vi "AlliGator Phasor Plot ROI Manager.vi"() -> ()   [LabVIEW 2021, in "AlliGator ROIs.lvlib"]
doc: "Phasor Plot image ROI list display UI."
uses:
  AlliGator ROIs.lvlib
  AlliGator ROI Manager Actions.ctl
  AlliGator Refnums List.ctl
  Image/Image Control Refnum.ctl
  Image/Image Display Event.ctl
  <vilib>/Utility/miscctls.llb/LVPoint32TypeDef.ctl
  AlliGator Variables List.ctl
  Image/Named ROI Description.ctl
  Variant/Variant to Data/Variant to String.vi
  AlliGator Phasor Plot Image ROI Storage [SGL] v3.vi
  AlliGator Globals, Variables & Constants.lvlib
  Image/Image.lvlib
  AlliGator Action Engine.lvlib
  Notebook/Notebook.lvlib
  AlliGator Notebook.lvlib
  Variant/Variant to Data/Variant to Data.lvlib
  AlliGator Phasor Plot.lvlib
  Rich Text Box/Rich Text Box.lvlib
panel:
  in  "ROI List":i32(listbox)
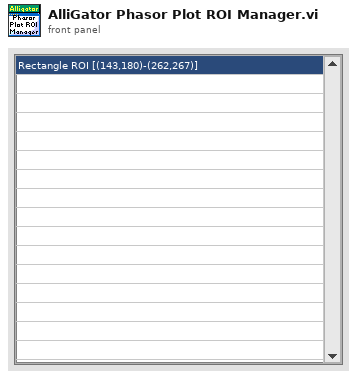
[diagram p1: front panel]
types:
  T1 = typedef "Image.lvlib/Image Control Refnum.ctl" = refnum<vi>
  T2 = typedef "AlliGator Globals, Variables & Constants.lvlib/AlliGator Refnums List.ctl" = enum16{"---------- AlliGator Controls ----------", "AlliGator Tab Control Refnum", "---------- AlliGator Indicators ----------", "Source Image Display Refnum", "Phasor Plot Display Refnum", "Decay Fit Parameter Map Refnum", "---------- AlliGator VIs ----------", "AlliGator Settings Refnum", "AlliGator Launcher Refnum"}
  T3 = typedef "AlliGator ROIs.lvlib/AlliGator ROI Manager Actions.ctl" = enum16{"Undefined", "Delete Current ROI", "Delete All Unselected ROIs", "Delete Multiple ROIs", "Delete All ROIs", "Swap ROIs", "Insert ROI", "Update Current ROI Descriptor", "Rename Current ROI", "Store New ROI", "Store Multiple ROIs", "Select Next ROI", "Select Previous ROI", "Find Selected ROI", "Show All ROIs", "Update ROI Manager Window", "Merge All ROIs", "Unmerge ROI", "Set Selected ROI by ID"}
  T4 = typedef "AlliGator ROIs.lvlib/AlliGator Image ROI Event refnum.ctl" = refnum<user-event>
  T5 = typedef "ROI Descriptor" = cluster{"Global Rectangle":i32[], "Contours":cluster{"ID":enum32{"External", "Internal"}, "Type":u32, "Coordinates":i32[]}[]}
  T6 = typedef "Image.lvlib/Image Display Event.ctl" = cluster{"Item Tag":string, "Image Control Refnum":T1, "Coords":T7, "Item Path":string}
  T7 = typedef "LVPoint32TypeDef.ctl" = cluster{"Horizontal":i32, "Vertical":i32}
  T8 = typedef "AlliGator Globals, Variables & Constants.lvlib/AlliGator Variables List.ctl" = enum16{"---- GUI ----", "Initialization Status", "State Indicators Refnum", "Original AlliGator Menu Items", "Current Action Loop State", "Script in progress", "Playback", "Loop Playback", "Search ROI Used", "Search ROI", "Decay Graph Max Legend Size", "Intensity Graph Max Legend Size", "Decay Statistics Graph Max Legend Size", "Phasor Graph Max Legend Size", "Phasor Ratio Graph Max Legend Size", "Lifetime Graph Max Legend Size", "---- Files ----", "Export Dataset Frames as Individual Files", "Show Batch Export Help Balloons", "Frames in Dataset", "ptu File Frame Start Indices", "Current Frame in Dataset", "Current Frame Timestamp", "------ Python Plugins ------", "Python Plugins Information", "Python Session", "Valid Python Session?", "---- Source Image ----", "Dataset Loaded", "Dataset Metadata", "Dataset Channel", "Dataset Data Description", "Background Dataset Metadata", "Background Dataset Channel", "Background Dataset Data Description", "Background File Subtraction", "Background File Path", "Background File Pile-up Correction", "Background File Pixel Well Capacity", "Background File Scaling Factor", "Source Image ROIs", "Current Source Image ROI", "Source Image ROI Event Refnum", "X_Source Image Display Range", "X_Source Image Palette Information", "Source Image Palette List", "Source Image Scale", "Current Dataset Load Settings", "Source Image:ROI Overlay Color", "---- Image Profile Window ----", "Image Profile:Overlay ROI in Source Image", "Image Profile Window Event Refnum", "Image Profile:IntensityType", "Image Profile:Intensity Average Type", "Image Profile:Intensity-weighted SDV", "Image Profile:Box Profile Type", "Image Profile Window Open", "Image Profile:Plotted Fit Parameter", "X_Type of Displayed Image", "X_Time Gate Slider", "Dataset Path", "Source Image Overlay to Erase", "Is Displayed Image Accumulated", "White Light Image Modified", "Mask Image Modified", "Macrotime Gate Separation", "------ Phasor Graph -------", "Phasor Graph:Show Line", "---- Phasor Plot ---", "Phasor Plot Parameters Changed", "FLI Dataset Modified since last Phasor Plot Calculation", "Phasor Harmonics Data", "Selected Phasor Harmonics", "Phasor Harmonic Manager Event Refnum", "Phasor Plot ROIs", "Current Phasor Plot ROI", "Phasor Plot ROI Event Refnum", "Phasor Plot Image Reference Points", "Phasor Plot Computed", "Phasor Plot Palette Information", "Phasor Plot Palette List", "Phasor Ratio Palette Information", "Phasor Ratio Palette List", "Phasor Image Scale", "Phasor Plot Image Overlay to Erase", "Phasor Plot Image Elements to Update", "Current Phasor Plot Calculation Parameters", "Current Phasor Calibration Options", "Reset Cumulated Phasor Plot", "Phasor Ratio Reference 1", "Phasor Ratio Lifetime Reference 1", "Phasor Ratio Reference 1 Frequency", "Phasor Ratio Reference 2", "Phasor Ratio Lifetime Reference 2", "Phasor Ratio Reference 2 Frequency", "---- Decay Analysis ----", "Number of Selected Decays to Fit", "LS Fit Results", "LAR Fit Results", "BS Fit Results", "Last Decay Max - Min", "Best Fit Parameters", "Best Fit Parameter Names", "Actual Size X", "Actual Size Y", "Binning X", "Binning Y", "Actual # Gates", "Dataset Number", "Gates to...", "Gates Skipped", "Gates to keep", "Gate Step", "Gate Separation", "Reversed Gates", "Pile-up Correction", "Pixel Well Capacity", "Background Subtracted", "Background Subtraction Method", "Background Definition Range", "Background File (deprecated)", "Number of Dataset Accumulated", "Array of Accumulated Dataset Paths", "Do Averaged Datasets", "Destination File Path", "Process Plot Target", "Use 1/D as Phasor Frequency", "---- Decay Fit Parameter Map -----", "Decay Fit Parameter Map Palette Information", "Decay Fit Parameter Map Palette List", "Local Decay Graph Window Event Refnum", "------- Local Decay Window ---------", "Use normalized IRF for convolution", "----- Miscellaneous ----", "Skippable Dialog Windows Status"}
  T9 = typedef "Image.lvlib/Named ROI Description.ctl" = cluster{"ROI Descriptor":T5, "ROI Name":string, "Overlay Color":u32}
  T10 = cluster{"data name":string, "drag data":variant}[]
  T11 = typedef "AlliGator Action Engine.lvlib/AlliGator Q Element.ctl" = cluster{"AlliGator Q Event":T12, "Data":variant}
  T12 = typedef "AlliGator Action Engine.lvlib/AlliGator Q Event.ctl" = enum16{"---- Files ----", "Files:Set Batch Export Files To Save", "Files:Set Dataset Loading & Pre-processing Options", "Files:Check #Frames in Dataset", "Files:Increment Frame Index", "Files:Open Mask Image", "Files:Open White Light Image", "Files:Open Single Dataset", "Files:New Folder of Folders Selected", "Files:Load File (all Types)_Scriptable", "Files:Move Flattened Series to Folders Series", "Files:Select Folder", "Files:Load FLI Dataset", "Files:Load Swiss SPAD 1 Dataset", "Files:Load Swiss SPAD 2 Dataset", "Files:Load .sdt FLI Dataset", "Files:Load .ptu FLI Dataset", "Files:Load .bin FLI Dataset", "Files:Load Single Gate Image Folder", "Files:Load I/m/phi Dataset (deprecated)", "Files:Load Single Image", "Files:Subtract Background File", "Files:Export FLI Dataset", "Files:Load HDF5 FLI Dataset", "Files:Set Destination File Path", "Files:Save Mask Image", "Files:Batch Conversion", "Files:New Folder Selected", "Files:Close FLI Dataset", "Files:Close FLI Dataset Series", "Files:Close White Light Image", "Files:Close Mask Image", "---- FLI Dataset ----", "FLI Dataset:Channel Arithmetic", "FLI Dataset:Export Average Lifetime Map as ASCII", "FLI Dataset:Export User-Defined Quantity Map as ASCII", "FLI Dataset:Python Function FLI Dataset Event", "FLI Dataset:ROI Analysis", "FLI Dataset:Tilted Logistic Square Gated IRF Characteristics Map", "FLI Dataset:Logistic Square Gated IRF Characteristics Map", "FLI Dataset:Square Gated IRF Characteristics Map", "FLI Dataset:Multi-ROI Single-Pixel Phasor Analysis", "FLI Dataset:Multi-ROI Single-Pixel NLSF Analysis", "FLI Dataset:All ROIs IRF Extraction", "FLI Dataset:All ROIs Decay Fit Non-Interactive (Fast + Individual IRF)", "FLI Dataset:All ROIs Phasor Analysis", "FLI Dataset:All ROIs Decay Fit", "FLI Dataset:Fluorescence Decay Statistics", "FLI Dataset:Update Decay Statistics Graph", "FLI Dataset:Get Decay from ROI", "FLI Dataset:All ROIs Average Lifetimes", "---- FLI Dataset Series ----", "FLI Dataset Series:Sum All Datasets in Series", "FLI Dataset Series:Add Dataset to Accumulated Dataset", "FLI Dataset Series:Display Accumulated Dataset", "FLI Dataset Series:Clear Dataset Series Sum", "FLI Dataset Series:Time-Series Analysis (NLSF)", "FLI Dataset Series:Time-Series Analysis (Phasor)", "---- Image ----", "Image:Update Image Profile Plots", "Image:Image Histogram Cursor Move", "Image:Image Histogram", "Image:Image Contrast", "Image:Set Image Histogram Cursor Move Flag", "Image:Clear Image Overlay", "Image:Use ROI as Search Area", "Image:Set ROI Diameter", "Image:Save Image Data as TIFF", "Image:Save Displayed Image with Overlay", "Image:Save Image Overlay Only", "Image:Save Image as Hot Pixel Mask", "Image:Change Source Image Color Palette", "Image:Copy Image to Clipboard", "Image:Source Image ROI Selection", "Image:Delete All ROIs", "Image:Delete All Unselected ROIs", "Image:Delete ROI", "Image:Merge All ROIs", "Image:Store ROI", "Image:Source Image ROI Storage", "Image:Export ROI Description to Notebook", "Image:Save ROI", "Image:Load ROI", "Image:Paste ROI Definition", "Image:Clear ROI", "Image:Identify ROIs in Mask Image", "Image:Create Complementary ROI", "Image:Create Contour ROI", "Image:Create ROI(s) from Pixels with Peak above Min_Scriptable", "Image:Create ROI(s) from Pixels with Intensity above Min_Scriptable", "Image:Compute ROI Statistics", "Image:Delete ROI(s) based on ROI Characteristics", "Image:Create ROI Grid", "Image:ROI to Individual Pixel ROIs", "Image:Python Function Source Image Event", "Image:Show Phasor Calibration Map ROI Centers", "Image:Convert ROI to Mask Image", "Image:Mouse Move", "Image:Mouse Up", "Image:Set Source Image Mouse Move Flag", "Image:Add Scale Bar Overlay", "Image:Delete Existing ROIs Option", "---- Decay ----", "Decay:Clear IRF/Reference Plot", "Decay:Clear Local IRFs", "Decay:Add Decay to Graph", "Decay:Smoothen Plot", "Decay:Smoothen Plot Tail", "Decay:Average Selected Plots", "Decay:Extract IRF", "Decay:Optimal IRF Extraction", "Decay:Threshold IRF", "Decay:Fit to Model IRF", "Decay:Fit IRF to Square Gate", "Decay:Fit IRF to Logistic Square Gate", "Decay:Fit IRF to Tilted Logistic Square Gate", "Decay:Create Bounding Cursors Set", "Decay:Export Bounding Cursors Definition to Notebook", "Decay:Denoise Plot", "Decay:Compute Cumulative Function", "Decay:Use as Reference Decay", "Decay:Show Reference Decay/IRF", "Decay:Extrapolate Decay", "Decay:Create Head & Tail Bounding Cursors", "Decay:Store Cursor-defined Head & Tail Fractions", "Decay:Rebin Plot", "Decay:1-Normalize Decay", "Decay:[0-1]-Normalize Plot", "Decay:Straighten Decay", "Decay:Shift Decay", "Decay:Fold Decay", "Decay:Fit Decay", "Decay:Global Fit of Selected Decays", "Decay:Post Global Fit Script", "Decay:Add Global Fit Parameters to Graph", "Decay:Add Decay Parameter(s) to Plot (Graph)", "Decay:Export Decay to Phasor Graph", "Decay:Plot Decay Shifts", "Decay:Compute Average Lifetime", "Decay:Plot Convolution", "Decay:Graph Tip Strip Update", "---- Decay Statistics ----", "Decay Statistics:Tip Strip Update", "---- Intensity Time Trace ----", "Intensity Time Trace:Use File Timestamp", "Intensity Time Trace:Load Intensity Corrections File", "Intensity Time Trace:Clear Intensity Corrections File", "Intensity Time Trace:Tip Strip Update", "---- Phasor Plot ----", "Phasor Plot:Build Phasor Plot", "Phasor Plot:Change Phasor Plot Color Palette", "Phasor Plot:Adjust Phasor Plot Display Range", "Phasor Plot:Highlight Image ROI in Phasor Plot", "Phasor Plot:Save Phasor Plot Image with Overlay", "Phasor Plot:Export Complex Phasor Map", "Phasor Plot:Export Phasor Ratio Map", "Phasor Plot:Export Average Lifetime Map", "Phasor Plot:Compute Phase Lifetime Histogram", "Phasor Plot:Compute Phasor Ratio Histogram", "Phasor Plot:Compute Phase Lifetime vs Intensity Scatter Plot", "Phasor Plot:Weber 2-Component Decomposition", "Phasor Plot:Update Phasor Color Map Vertices", "Phasor Plot:Clear Phasor Overlay", "Phasor Plot:Use Segment Extremities as References", "Phasor Plot:Use UC/Segment Intersections as References", "Phasor Plot:Use UC/Principal Axis Intersections as References", "Phasor Plot:Use UC/Linear Fit Intersections as References", "Phasor Plot:Update Phasor Plot Reference", "Phasor Plot:Show Local Phasor Info in Phasor Plot", "Phasor Plot:Update Phasor Plot State", "Phasor Plot:Phasor Plot ROI Storage", "Phasor Plot:Phasor Plot ROI Selection", "Phasor Plot:Python Function Phasor Plot Event", "Phasor Plot:Overlay Phasor ROI, Ratio or Map in Source Image", "Phasor Plot:Compute Decay of Selected Phasors", "Phasor Plot:Phasor at Image Pixel", "Phasor Plot:Mouse Move", "Phasor Plot:Mouse Up", "Phasor Plot:Display Range Mouse Move", "Phasor Plot:Set Mouse Move Flag", "---- Phasor Graph ----", "Phasor Graph:Calibrated Phasor Map Series", "Phasor Graph:Whole Image Phasor Scatter Plot (Todo)", "Phasor Graph:Get Phasor Value", "Phasor Graph:Create New Phasor Plot Dialog", "Phasor Graph:Update Last Phasor Value", "Phasor Graph:Update Phasor (m, phi)", "Phasor Graph:Remove Single Phasor from Plot", "Phasor Graph:Add Single Phasor to Plot", "Phasor Graph:Remove Phasor Plot", "Phasor Graph:Remove Selected Phasor Plots", "Phasor Graph:Clear Phasor Data", "Phasor Graph:Clear Phasor Graph", "Phasor Graph:Cursor Move", "Phasor Graph:Draw Cursor Connecting Line", "Phasor Graph:Clear Cursor Connecting Line", "Phasor Graph:Find UC Intersection", "Phasor Graph:Use UC/Cursor-Defined Line Intersections", "Phasor Graph:Use Selected Plots Fitted Line/UC Intersections", "Phasor Graph:Use Selected Plots Principal Axis/UC Intersections", "Phasor Graph:Show Single Phasor", "Phasor Graph:Save Single Phasor Plot", "Phasor Graph:Save All Phasor Plots", "Phasor Graph:Load Phasor Plot(s)", "Phasor Graph:Phasor Multiplication", "Phasor Graph:Compute Average Phasor", "Phasor Graph:Compute Multiple Average Phasors (Selected Plots)", "Phasor Graph:Export Single Phasor Plot Phase Lifetimes", "Phasor Graph:Phase Lifetime Trajectory", "Phasor Graph:Phase Lifetime vs Intensity Scatter Plot (deprecated)", "Phasor Graph:Parameter 2 vs Parameter 1 Scatter Plot", "Phasor Graph:Use Cursor n Location", "Phasor Graph:Set Reference n to Current Phase Lifetime Value", "Phasor Graph:Set Reference n to Lifetime Value", "Phasor Graph:Set Cursor n Location", "Phasor Graph:Save Phasor Graph Image", "Phasor Graph:Update SEPL Plot", "Phasor Graph:Export Single Phasor Plot Data", "Phasor Graph:Export Selected Phasor Plots Data", "Phasor Graph:Python Function Phasor Graph Event", "Phasor Graph:Tip Strip Update", "---- Calibration ----", "Calibration:Set Calibration Type", "Calibration:Load/Save Phasor Calibration", "Calibration:Load/Save Phasor Calibration Series", "Calibration:Load/Save Phasor Calibration Map", "Calibration:Use as Calibration", "Calibration:Compute Optimal Calibration from Phasor References", "Calibration:Clear Phasor Calibration", "Calibration:Single Phasor Calibration Information", "Calibration:Use as Calibration Series", "Calibration:Use as Calibration Map", "Calibration:Clear Calibration Series", "Calibration:Phasor Calibration Series Information", "Calibration:Clear Calibration Map", "Calibration:Phasor Calibration Map Information", "Calibration:Apply Phasor Calibration", "Calibration:Update Single Plot Calibration", "Calibration:Update Multiple Plots Calibration", "Calibration:Clear Single Plot Calibration", "Calibration:Clear All Plots Calibrations", "Calibration:Clear Plot(s) Calibration(s)?", "Calibration:Phasor Calibration Maps (# Gates Series)", "---- Phasor Ratio ----", "Phasor Ratio:Clear Reference n", "Phasor Ratio:Toggle Selected Plot(s)  Lock to Reference 1", "Phasor Ratio:Use as Reference n", "Phasor Ratio:Send Reference n to Notebook", "Phasor Ratio:Toggle Selected Plot(s)  Lock to Reference 2", "Phasor Ratio:Compute Phasor Ratio at Mouse Location", "Phasor Ratio:Compute Phasor Plot's Average Phasor Ratio", "Phasor Ratio:Compute Time-Series Phasor Ratios", "Phasor Ratio:Fit Line to Phasor Ratio Plot", "Phasor Ratio:Save References", "Phasor Ratio:Load References", "Phasor Ratio:Update Phasor Reference 1", "Phasor Ratio:Update Phasor Reference 2", "Phasor Ratio:Move Cursor n to Reference n", "Phasor Ratio:Use as Phasor Reference 1 Lifetime", "Phasor Ratio:Use as Phasor Reference 2 Lifetime", "Phasor Ratio:Export Phasor Ratio Map as ASCII", "Phasor Ratio:Tip Strip Update", "---- Lifetime & Other Parameters Graph ----", "Lifetime:Tip Strip Update", "---- Decay Fit Parameter Map ----", "Decay Fit Parameter Map:Export ROI NLSF Data as ASCII", "Decay Fit Parameter Map:Set Decay Fit  Parameter Map Selection", "Decay Fit Parameter Map:Build Decay Fit Parameter Map", "Decay Fit Parameter Map:Change Decay Fit Parameter Map Color Palette", "Decay Fit Parameter Map:Export Decay Fit Parameter Map Data as ASCII", "Decay Fit Parameter Map:Export All Decay Fit Parameter Maps Data as ASCII", "Decay Fit Parameter Map:Send Map Data to Lifetime Graph", "Decay Fit Parameter Map:Save Decay Fit Parameter Map Image", "Decay Fit Parameter Map:Save-Load IRFs & Fit Data", "Decay Fit Parameter Map:Update Local Decay Plots", "Decay Fit Parameter Map:Python Function Decay Fit Parameters Map Event", "Decay Fit Parameter Map:Overlay Decay Fit Parameter Map in Source Image", "Decay Fit Parameter Map:Plot Map Data vs Intensity", "Decay Fit Parameter Map:Mouse Up", "Decay Fit Parameter Map:Display Range Mouse Move", "---- Generic Graph ----", "Generic Graph:Generic XY Graph Event", "Generic Graph:Python Function XY Graph Event", "Generic Graph:New Plot", "Generic Graph:Save Plot", "Generic Graph:XY Plot Histogram", "Generic Graph:Set XY Graph Plot Name", "Generic Graph:Set Last Cursor Style", "Generic Graph:Tip Strip Update", "---- GUI ----", "GUI:Start Script", "GUI:Type of Displayed Image Changed", "GUI:Gate Image Slide Changed", "GUI:Show Busy Icon", "GUI:Show Busy Icon & Abort Button", "GUI:Hide Busy Icon", "GUI:Hide Busy Icon & Abort Button", "GUI:Abort", "GUI:End Script", "GUI:Start Timing", "GUI:End Timing", "GUI:Set State Indicator", "GUI:Send Parameters JSON Strings to Clipboard", "GUI:Set Gate Step", "GUI:Idle", "GUI:Initialization", "GUI:Quit", "GUI:Increment Dataset Index", "GUI:Set Dataset Index to -1", "GUI:Time Series Slider Moved", "GUI:Time Series Slider Changed", "GUI:Toggle Playback or Loop", "GUI:Playback Script", "GUI:Set Phasor Frequency", "GUI:Open Window", "GUI:Start Test Script", "GUI:End Test Script", "DEBUG"}
  T13 = typedef "Rich Text Box.lvlib/Text Formatting.ctl" = cluster{"Font":string, "Text Color":T14, "Text Background Color":T14, "Text Style":enum16{"Regular", "Bold", "Italic", "Underline", "Strikeout"}, "Font Size (Points)":dbl, "Text Alignment":i32}
  T14 = typedef "Rich Text Box.lvlib/Text Colors.ctl" = enum16{"Unchanged", "Black", "Blue", "Brown", "Gray", "Green", "Orange", "Pink", "Red", "White"}
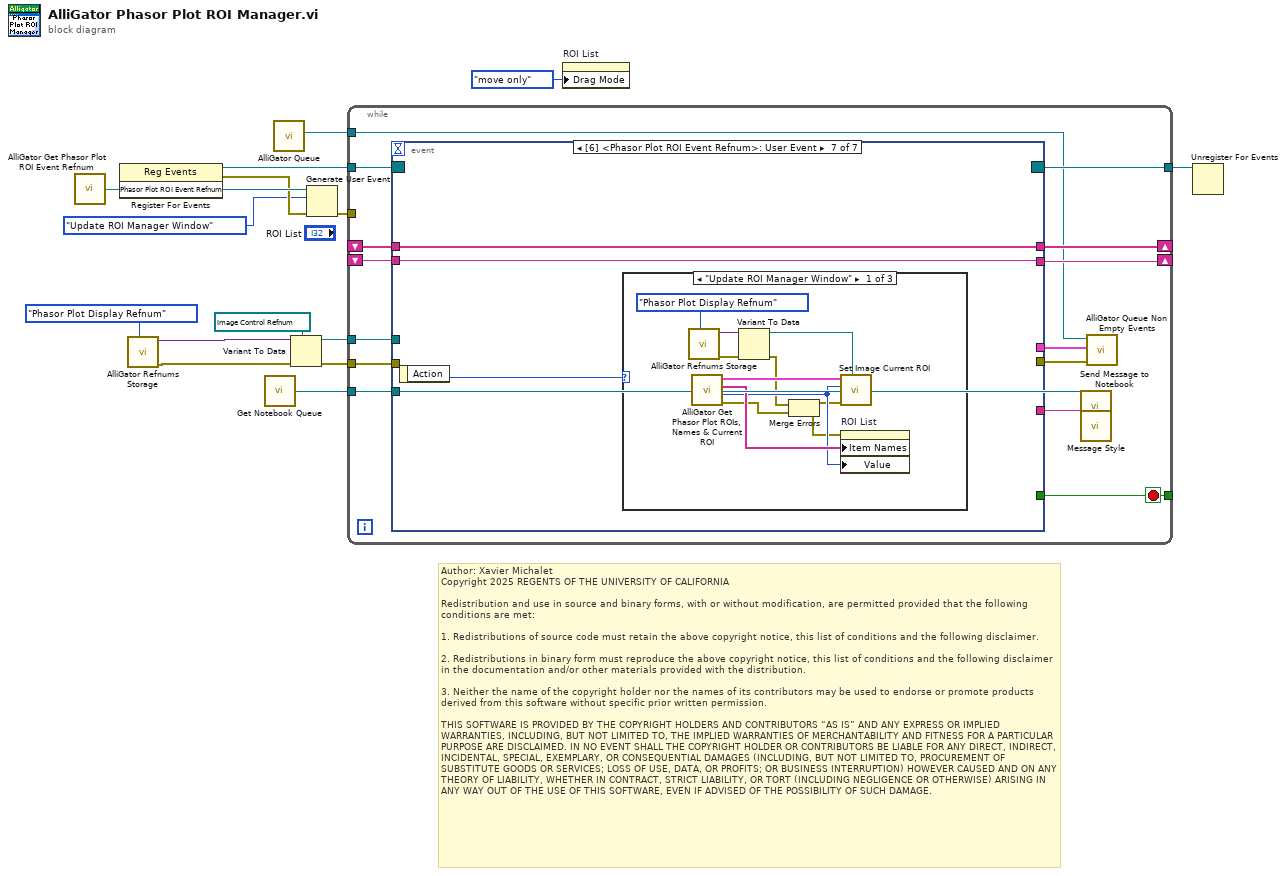
[diagram p0: block diagram]
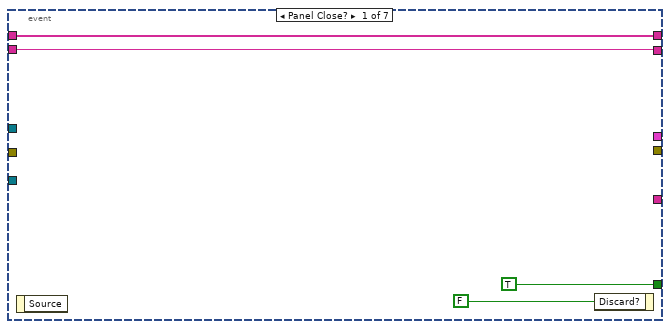
[diagram p2: hidden frame]
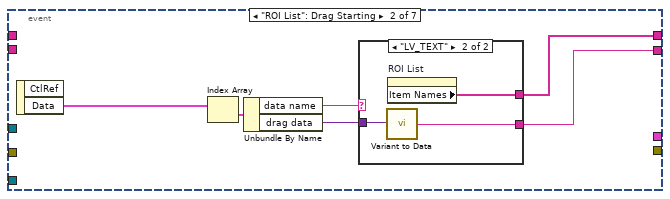
[diagram p3: hidden frame]
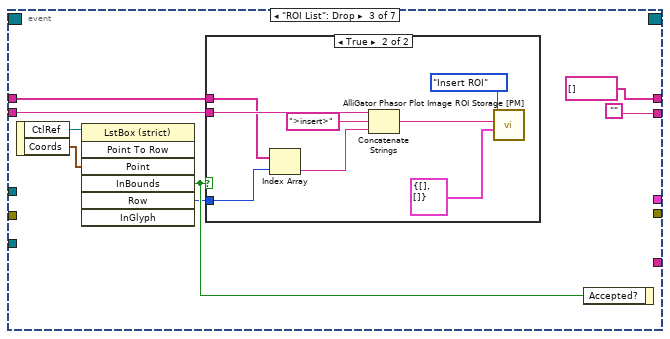
[diagram p5: hidden frame]
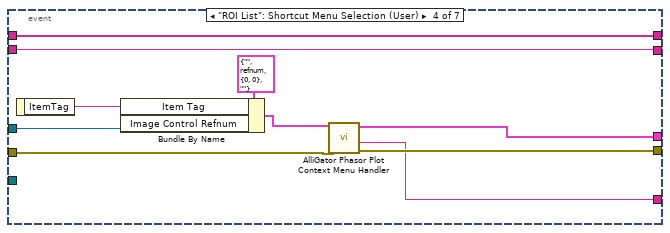
[diagram p7: hidden frame]
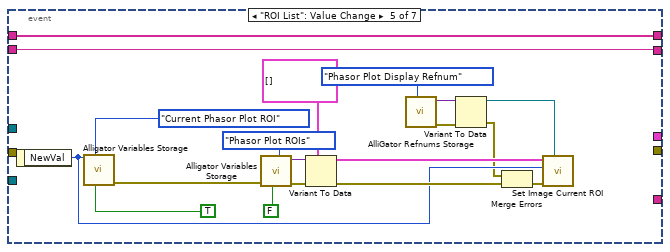
[diagram p8: hidden frame]
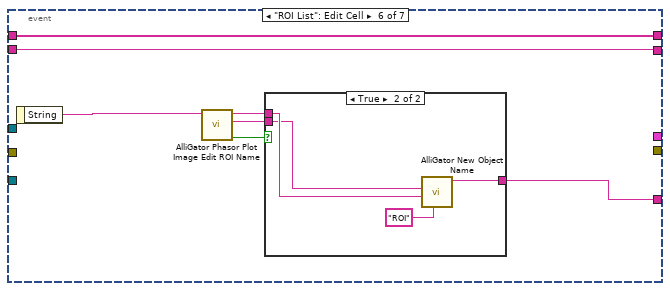
[diagram p9: hidden frame]
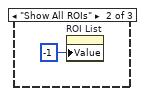
[diagram p11: hidden frame]
diagram:
  # "Author: Xavier Michalet\nCopyright 2025 REGENTS OF THE UNIVERSITY OF CALIFORNIA\n\nRedistribution and use in source and binary forms, with or without modification, are permitted provided that the following conditions are met:\n\n1. Redistributions of source code must retain the above copyright notice, this list of conditions and the following disclaimer.\n\n2. Redistributions in binary form must reproduce the above copyright notice, this list of conditions and the following disclaimer in the documentation and/or other materials provided with the distribution.\n\n3. Neither the name of the copyright holder nor the names of its contributors may be used to endorse or promote products derived from this software without specific prior written permission.\n\nTHIS SOFTWARE IS PROVIDED BY THE COPYRIGHT HOLDERS AND CONTRIBUTORS “AS IS” AND ANY EXPRESS OR IMPLIED WARRANTIES, INCLUDING, BUT NOT LIMITED TO, THE IMPLIED WARRANTIES OF MERCHANTABILITY AND FITNESS FOR A PARTICULAR PURPOSE ARE DISCLAIMED. IN NO EVENT SHALL THE COPYRIGHT HOLDER OR CONTRIBUTORS BE LIABLE FOR ANY DIRECT, INDIRECT, INCIDENTAL, SPECIAL, EXEMPLARY, OR CONSEQUENTIAL DAMAGES (INCLUDING, BUT NOT LIMITED TO, PROCUREMENT OF SUBSTITUTE GOODS OR SERVICES; LOSS OF USE, DATA, OR PROFITS; OR BUSINESS INTERRUPTION) HOWEVER CAUSED AND ON ANY THEORY OF LIABILITY, WHETHER IN CONTRACT, STRICT LIABILITY, OR TORT (INCLUDING NEGLIGENCE OR OTHERWISE) ARISING IN ANY WAY OUT OF THE USE OF THIS SOFTWARE, EVEN IF ADVISED OF THE POSSIBILITY OF SUCH DAMAGE."
  n1 = call "AlliGator Get Phasor Plot ROI Event Refnum.vi"() -> ("Phasor Plot ROI Event Refnum"=w11:T4)
  n2 = register-events(w11) -> (reference out=w15:refnum<event-registration>, error out=w10:errorcluster)  [unwired: 2 in]
  n3 = call "AlliGator Refnums Storage.vi"("AlliGator Refnum List"=AlliGator_Refnums_List."Phasor Plot Display Refnum") -> ("Error Out"=w1:errorcluster, "Data out"=w6:variant)  [unwired: 9 in]
  n4 = call "Get Notebook Queue.vi"() -> ("Notebook Queue"=w12:refnum<queue>)  [unwired: 9 in]
  n5 = call "AlliGator Queue.vi"() -> ("AlliGator Q"=w13:refnum<queue>)  [unwired: 8 in, 1 out]
  n6 = Variant To Data(error in=w1, type=T1 refnum ("Image Control Refnum"), Variant=w6) -> (data=w3:T1, error out=w4:errorcluster)
  n7 = Generate User Event(user event=w11, event data cluster=AlliGator_ROI_Manager_Actions."Update ROI Manager Window" ("event data"), error in=w10) -> (error out=w9:errorcluster)  [unwired: 1 in, 1 out]
  n8 = while {
    tunnel: w15 -> [w30]
    tunnel: [w29] -> w14
    tunnel: w13 -> [w20]
    tunnel: w12 -> [w17]
    shift-right: [w28] -> _
    shift-left: _ -> [w27]
    shift-right: [w26] -> _
    shift-left: _ -> [w25]
    tunnel: w9 -> [_]
    tunnel: [w24] -> _
    tunnel: w4 -> [w23]
    tunnel: w3 -> [w22]
    stop <- w24 stop-if-true
    n9 = event shown="[6] <Phasor Plot ROI Event Refnum>: User Event" {
      selector: w30 -> [_ _ _ _ _ _ _]
      dyn-events: [_ _ _ _ _ _ _] -> w29
      timeout: _ -> [_ _ _ _ _ _ _]
      tunnel: [TRUE _ _ _ _ _ _] -> w24
      tunnel: w17 -> [_ _ _ _ _ _ _]
      tunnel: [w32 w37 "" w69 w77 w91 w102] -> w28
      tunnel: w27 -> [w32 _ w51 w69 w77 w91 w102]
      tunnel: [w31 w35 string[] [] ("Item Names") w68 w76 w90 w101] -> w26
      tunnel: w25 -> [w31 _ w49 w68 w76 w90 w101]
      tunnel: w23 -> [_ _ _ w67 _ _ _]
      tunnel: w22 -> [_ _ _ w62 _ _ _]
      tunnel: [_ _ _ w66 _ _ _] -> w21
      tunnel: [_ _ _ w61 _ _ _] -> w19
      tunnel: [_ _ _ w60 _ w89 _] -> w16
      event Panel Close? {
        n10 = event-data() -> ()  [unwired: 1 in, 1 out]
        n11 = event-data("Discard?"=FALSE) -> ()  [unwired: 1 in, 1 out]
      }
      event "ROI List": Drag Starting {
        n12 = event-data() -> ("Data"=w40:T10)  [unwired: 1 in, 1 out]
        n13 = Index Array(array=w40) -> (element=w39:cluster{"data name":string, "drag data":variant})  [unwired: 1 in]
        n14 = Unbundle By Name(w39) -> ("data name"=w38:string, "drag data"=w36:variant)
        n15 = case shown="\"LV_TEXT\"" w38 {
          tunnel: [_ w42] -> w37
          tunnel: w36 -> [_ w43]
          tunnel: [_ w41] -> w35
          frame "False", Default {
          }
          frame "LV_TEXT" {
            n16 = call-poly "Variant to Data.vi"("Variant"=w43) -> ("String"=w42:string)  [unwired: 8 in]
            n17 = property on="ROI List" class="LstBox (strict)"() -> ("Item Names"=w41:string[])  [unwired: 2 in, 2 out]
          }
        }
      }
      event "ROI List": Drop {
        n18 = event-data() -> ("CtlRef"=w47:refnum<vi>, "Coords"=w46:T7)  [unwired: 1 in]
        n19 = invoke class="LstBox (strict)" method="Point To Row"(reference=w47, "Point"=w46) -> ("InBounds"=w45:bool, "Row"=w44:i32)  [unwired: 5 in, 5 out]
        n20 = case shown="True" w45 {
          tunnel: w51 -> [_ w57]
          tunnel: w49 -> [_ w56]
          tunnel: w44 -> [_ w52]
          frame False {
          }
          frame True {
            n21 = Index Array(array=w56, index=w52) -> (element=w59:string)
            n22 = Concatenate Strings(w57, ">insert>" ("string"), w59) -> (w55:string)
            n23 = call-poly "AlliGator Phasor Plot Image ROI Storage [PM].vi"("Current ROI Descriptor"=T5 {"Global Rectangle"=[], "Contours"=[]}, "Default Name (\"ROI\")"=w55, "Action"=AlliGator_ROI_Manager_Actions."Insert ROI") -> ()  [unwired: 3 in, 6 out]
          }
        }
        n24 = event-data("Accepted?"=w45) -> ()  [unwired: 1 in, 1 out]
      }
      event "ROI List": Shortcut Menu Selection (User) {
        n25 = event-data() -> ("ItemTag"=w63:string)  [unwired: 1 in]
        n26 = Bundle By Name(cluster=T6 {"Item Tag"="", "Image Control Refnum"=refnum, "Coords"={"Horizontal"=0, "Vertical"=0}, "Item Path"=""} ("Image Event"), "Item Tag"=w63, "Image Control Refnum"=w62) -> (w65:T6)
        n27 = call "AlliGator Phasor Plot Context Menu Handler.vi"("Error In"=w67, "Image Event"=w65) -> ("Error Out"=w61:errorcluster, "Message"=w60:string, "AlliGator Actions"=w66:T11[])  [unwired: 7 in]
      }
      event "ROI List": Value Change {
        n28 = event-data() -> ("NewVal"=w78:i32)  [unwired: 1 in]
        n29 = call "Alligator Variables Storage.vi"("Get(F)/Set"=TRUE, "AlliGator Variable"=AlliGator_Variables_List."Current Phasor Plot ROI" ("Alligator Variable"), "Data in"=w78) -> ("Error Out"=w84:errorcluster)  [unwired: 6 in, 2 out]
        n30 = call "Alligator Variables Storage.vi"("Get(F)/Set"=FALSE, "AlliGator Variable"=AlliGator_Variables_List."Phasor Plot ROIs" ("Alligator Variable"), "Error In"=w84) -> ("Error Out"=w83:errorcluster, "Data out"=w86:variant)  [unwired: 6 in, 1 out]
        n31 = Variant To Data(error in=w83, type=T9[] [] ("Stored ROIs in"), Variant=w86) -> (data=w79:T9[], error out=w80:errorcluster)
        n32 = call "AlliGator Refnums Storage.vi"("AlliGator Refnum List"=AlliGator_Refnums_List."Phasor Plot Display Refnum") -> ("Error Out"=w75:errorcluster, "Data out"=w74:variant)  [unwired: 9 in]
        n33 = Variant To Data(error in=w75, Variant=w74) -> (data=w72:refnum<vi>, error out=w70:errorcluster)  [unwired: 1 in]
        n34 = Merge Errors(w70, w80) -> (w71:errorcluster)
        n35 = call "Set Image Current ROI.vi"("Image Refnum"=w72, "error in (no error)"=w71, "Current ROI"=w78, "Stored ROIs in"=w79) -> ()  [unwired: 7 in, 1 out]
      }
      event "ROI List": Edit Cell {
        n36 = event-data() -> ("String"=w95:string)  [unwired: 1 in]
        n37 = call "AlliGator Phasor Plot Image Edit ROI Name.vi"("ROI Name in"=w95) -> ("accepted?"=w93:bool, "Old ROI Name"=w92:string, "ROI Name out"=w94:string)  [unwired: 8 in]
        n38 = case shown="True" w93 {
          tunnel: w94 -> [_ w99]
          tunnel: w92 -> [_ w98]
          tunnel: [_ w96] -> w89
          frame False {
          }
          frame True {
            n39 = call "AlliGator New Object Name.vi"("Object String ('ROI')"="ROI", "Modified Object Name"=w99, "Original Object Name"=w98) -> ("Message"=w96:string)  [unwired: 7 in, 1 out]
          }
        }
      }
      event User Event {
        n40 = event-data() -> ("Action"=w100:T3)  [unwired: 1 in]
        n41 = case shown="\"Update ROI Manager Window\"" w100 {
          frame "Update ROI Manager Window" {
            n42 = call "AlliGator Refnums Storage.vi"("AlliGator Refnum List"=AlliGator_Refnums_List."Phasor Plot Display Refnum") -> ("Error Out"=w109:errorcluster, "Data out"=w108:variant)  [unwired: 9 in]
            n43 = call "AlliGator Get Phasor Plot ROIs, Names & Current ROI.vi"() -> ("Error Out"=w105:errorcluster, "Current ROI"=w110:i32, "ROI Names"=w111:string[], "Stored ROIs"=w112:T9[])  [unwired: 8 in]
            n44 = Variant To Data(error in=w109, Variant=w108) -> (data=w106:refnum<vi>, error out=w104:errorcluster)  [unwired: 1 in]
            n45 = Merge Errors(w104, w105) -> (w103:errorcluster)
            n46 = call "Set Image Current ROI.vi"("Image Refnum"=w106, "error in (no error)"=w103, "Current ROI"=w110, "Stored ROIs in"=w112) -> ()  [unwired: 7 in, 1 out]
            n47 = property on="ROI List" class="LstBox (strict)"(error in=w103, "Item Names"=w111, "Value"=w110) -> ()  [unwired: 1 in, 2 out]
          }
          frame "Show All ROIs" {
            n48 = property on="ROI List" class="LstBox (strict)"("Value"=-1 ("ROI List")) -> ()  [unwired: 2 in, 2 out]
          }
          frame Default {
          }
        }
      }
    }
    n49 = call "Message Style.vi"() -> ("Message Formatting"=w18:T13)
    n50 = call "Send Message to Notebook.vi"("Text Formatting"=w18, "Message"=w16, "Notebook Queue"=w17) -> ()  [unwired: 5 in, 2 out]
    n51 = call "AlliGator Queue Non Empty Events.vi"("Error In"=w19, "Actions"=w21, "AlliGator Q"=w20) -> ()  [unwired: 8 in, 1 out]
  }
  n52 = property on="ROI List" class="LstBox (strict)"("Drag Mode"=enum32{"copy or move", "copy only", "move only"}."move only" ("Drag/Drop:Drag Mode")) -> ()  [unwired: 2 in, 2 out]
  n53 = Unregister For Events(event registration refnum=w14) -> ()  [unwired: 1 in, 1 out]
